vi "Enqueue - State Command.vi"(7 "Insert?":bool=TRUE caption="Insert? (T)", 8 "error in (no error)":errorcluster, 9 "Data":T1=variant(string "Default"), 10 "Command":string, 11 "Queue in":T2) -> (0 "error out":errorcluster, 3 "Queue Out (dup)":T2)   [LabVIEW 2010]
doc: "This VI inserts a command into the queue appending \"State - \" to the Command field, with variant data.\n\nInputs:\nQueue in - queue reference (queue is cluster of Command (str) and Data (variant))\nCommand - (str) command to append to \"State - \" and insert into queue\nData - (variant) data to insert with command into queue\nInsert? - (bool) allows logic to be connected to determine if item should be inserted into the queue or skipped\nerror in - error input cluster\n\nOutputs:\nQueue out (dup) - duplicate of input queue reference\nerror out - error output cluster"
uses:
  <userlib>/Common/Queue with Cluster/TYP_Queue with Cluster Reference.ctl
  Controls/TYP_VariantDefault.ctl
  InternalState Command class/Internal State Command.lvclass
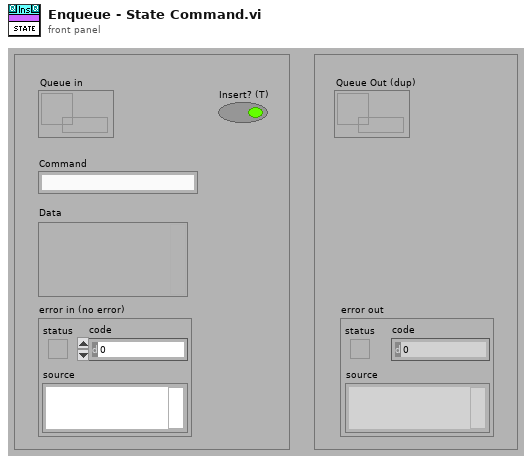
[diagram p1: front panel]
types:
  T1 = typedef "TYP_VariantDefault.ctl" = variant
  T2 = typedef "TYP_Queue with Cluster Reference.ctl" = refnum<queue>
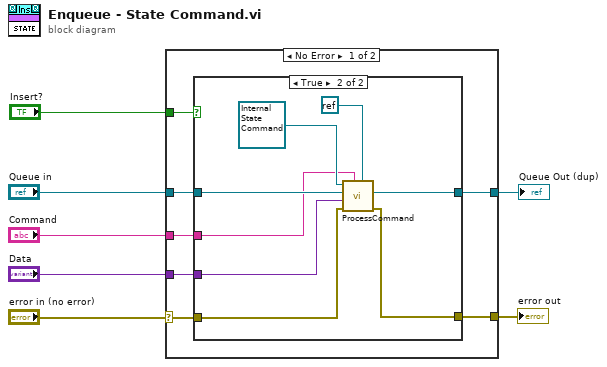
[diagram p0: block diagram]
diagram:
  n1 = case shown="No Error" "error in (no error)" {
    selector: "error in (no error)" -> [w9 w25]
    tunnel: "Queue in" -> [w14 w26]
    tunnel: [w13 w26] -> w6
    tunnel: "Data" -> [w12 _]
    tunnel: "Command" -> [w11 _]
    tunnel: [w10 w25] -> w3
    tunnel: "Insert?" -> [w8 _]
    frame No Error {
      n2 = case shown="True" w8 {
        tunnel: w14 -> [w15 w24]
        tunnel: [w15 w23] -> w13
        tunnel: w12 -> [_ w21]
        tunnel: w11 -> [_ w20]
        tunnel: [w16 w19] -> w10
        tunnel: w9 -> [w16 w18]
        frame False {
        }
        frame True {
          n3 = call-dynamic "ProcessCommand.vi"("Ctl Refnum"=refnum<k0> refnum, "Command"=w20, "error in (no error)"=w18, "Data"=w21, "Queue with Cluster Reference"=w24, "Internal State Command in"=refnum<class "Internal State Command.lvclass"> refnum ("Internal State Command.lvclass")) -> ("error out"=w19:errorcluster, "Queue (dup)"=w23:T2)  [unwired: 3 in, 1 out]
        }
      }
    }
    frame Error {
    }
  }
  "Queue Out (dup)" <- w6
  "error out" <- w3
